vi "getSize.vi"(8 "error in (no error)":errorcluster, 11 "Theme.Font in":refnum<class "Theme.Font.lvclass">) -> (0 "error out":errorcluster, 2 "Size":u32, 3 "Theme.Font out":refnum<class "Theme.Font.lvclass">)   [LabVIEW 2017, in "Theme.lvlib" / "Theme.Font.lvclass"]
uses:
  Theme.Font.lvclass
  Theme.Font.lvclass/Theme.Font.ctl
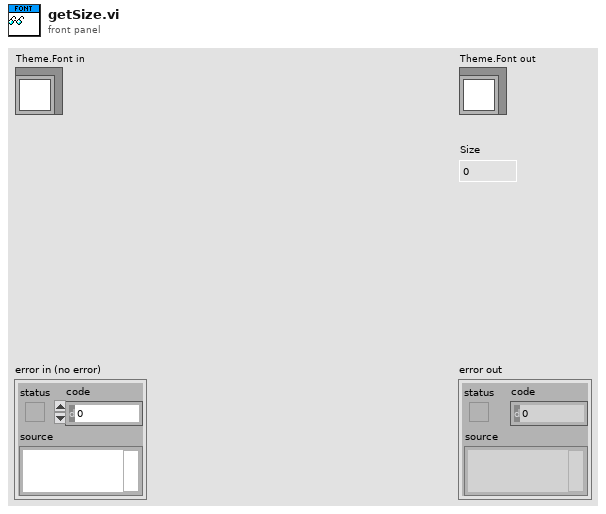
[diagram p1: front panel]
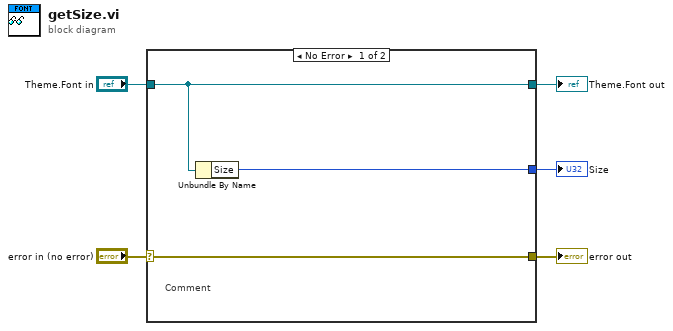
[diagram p0: block diagram]
diagram:
  n1 = case shown="No Error" "error in (no error)" {
    selector: "error in (no error)" -> [w8 w9]
    tunnel: [w8 w9] -> w4
    tunnel: [w7 w10] -> w2
    tunnel: "Theme.Font in" -> [w7 w10]
    tunnel: [w6 _] -> w1
    frame No Error {
      # "Comment"
      n2 = Unbundle By Name(w7) -> ("Size"=w6:u32)
    }
    frame Error {
    }
  }
  "error out" <- w4
  "Theme.Font out" <- w2
  "Size" <- w1
